vi "I2C Write Data.vi"(5 "Address":T2 format="%02x", 6 "NoStop (F)":bool, 7 "I2C #":T1=-1, 8 "error in (no error)":errorcluster, 10 "Data":string, 11 "DeviceComms in":refnum<class "DeviceComms.lvclass">) -> (0 "error out":errorcluster, 3 "DeviceComms out":refnum<class "DeviceComms.lvclass">)   [LabVIEW 2024, in "CTI.lvlib" / "DeviceComms.lvclass"]
uses:
  DeviceComms.lvclass
  I2C Address.ctl
  I2C Number.ctl
  CTI.lvlib
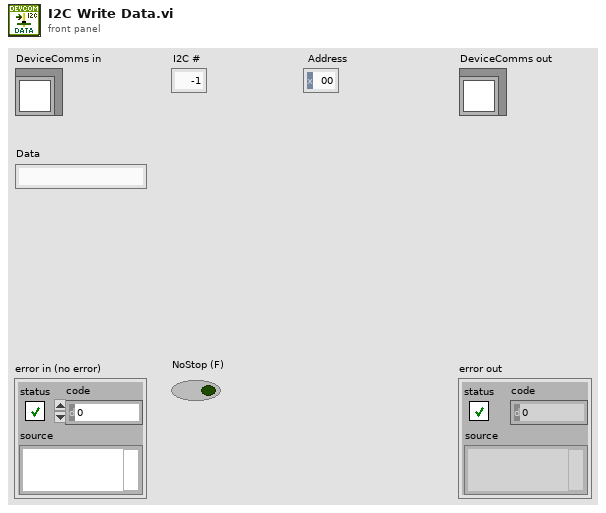
[diagram p1: front panel]
types:
  T1 = typedef "CTI.lvlib/I2C Number.ctl" = i8
  T2 = typedef "CTI.lvlib/I2C Address.ctl" = u8
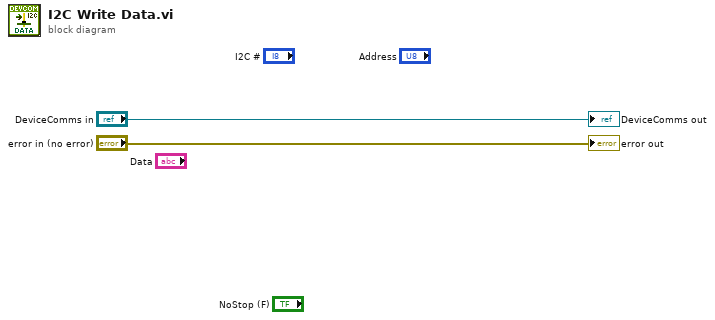
[diagram p0: block diagram]
diagram:
  "error out" <- "error in (no error)"
  "DeviceComms out" <- "DeviceComms in"
